vi "Set Position.vi"(8 "error in":errorcluster, 9 "Datum":T1, 10 "Target Coordinates":T2, 11 "Philips UI in":refnum<class "Flex UI.lvclass">) -> (0 "error out":errorcluster, 3 "Philips UI out":refnum<class "Flex UI.lvclass">)   [LabVIEW 2014, in "Flex UI.lvclass"]
doc: "Sets the position of the UI.\n\nThe Datum input specifies which part of the VI panel should be sent to those coordinates. For example, the Top-Left (corner) versus the Center point of the panel."
uses:
  Flex UI.lvclass
  <vilib>/Utility/miscctls.llb/LVPositionTypeDef.ctl
  Enum - Datum.ctl
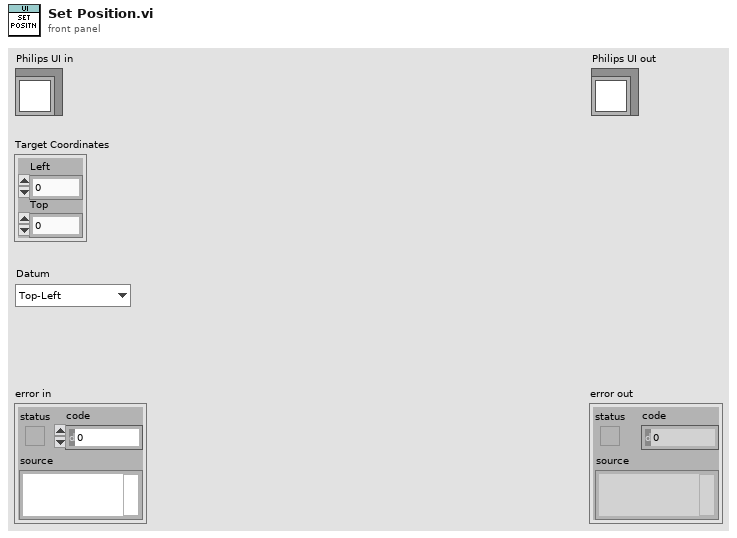
[diagram p1: front panel]
types:
  T1 = typedef "Flex UI.lvclass/Enum - Datum.ctl" = enum16{"Top-Left", "Top-Right", "Bottom-Left", "Bottom-Right", "Center"}
  T2 = typedef "LVPositionTypeDef.ctl" = cluster{"Left":i32, "Top":i32}
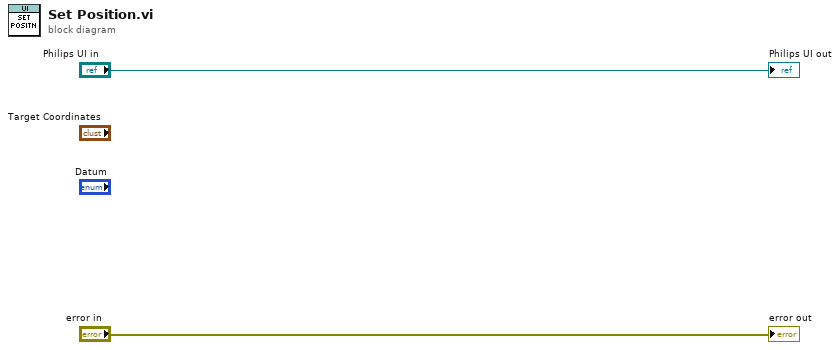
[diagram p0: block diagram]
diagram:
  "error out" <- "error in"
  "Philips UI out" <- "Philips UI in"
